vi "move-delayline-eventSD.vi"(3 "Delay pos (mm)":dbl, 4 "choix cible":u16(ring)=2 items=["definir position", "deplacer relatif", "deplacer absolu"], 6 "deplacement in":refnum<vi>) -> (0 "Delay (ps)":dbl=-0.0, 1 "moved":string, 2 "Delay (mm)":dbl, 5 "deplacement boolean":bool)   [LabVIEW 2015]
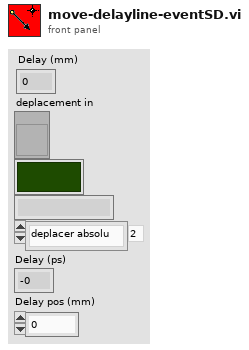
[diagram p1: front panel]
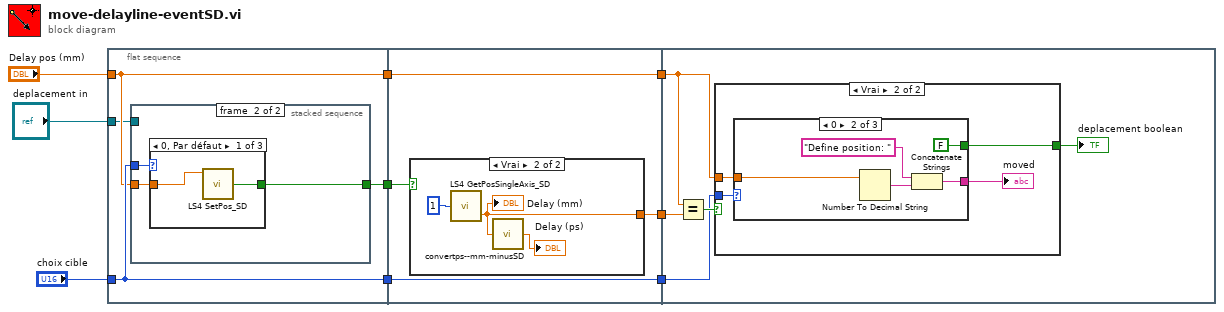
[diagram p0: block diagram]
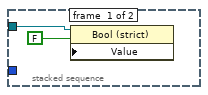
[diagram p2: hidden frame]
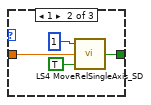
[diagram p3: hidden frame]
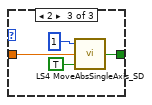
[diagram p4: hidden frame]
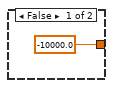
[diagram p5: hidden frame]
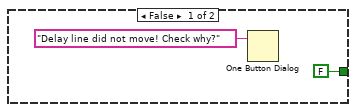
[diagram p6: hidden frame]
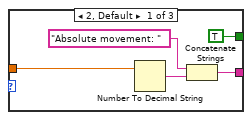
[diagram p7: hidden frame]
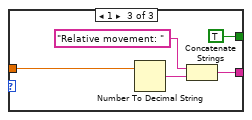
[diagram p8: hidden frame]
diagram:
  n1 = flat-sequence {
    tunnel: "choix cible" -> [w13]
    tunnel: [w13] -> w6
    tunnel: "Delay pos (mm)" -> [w12]
    tunnel: [w12] -> w5
    tunnel: "deplacement in" -> [w10]
    tunnel: [w11] -> w4
    tunnel: w6 -> [w30]
    tunnel: [w30] -> w3
    tunnel: w5 -> [w29]
    tunnel: [w29] -> w2
    tunnel: w4 -> [w32]
    tunnel: [w31] -> w1
    tunnel: w3 -> [w38]
    tunnel: w2 -> [w37]
    tunnel: w1 -> [w39]
    frame #0 {
      n2 = stacked-sequence {
        tunnel: [_ w18] -> w11
        tunnel: w12 -> [_ w17]
        tunnel: w13 -> [_ w16]
        tunnel: w10 -> [w14 _]
        frame #0 {
          n3 = property class="Bool (strict)"(reference=w14, "Value"=FALSE ("deplacement boolean")) -> ()  [unwired: 1 in, 2 out]
        }
        frame #1 {
          n4 = case "Structure Condition" shown="0, Par défaut" w16 {
            tunnel: w17 -> [w20 w22 w26]
            tunnel: [w19 w21 w25] -> w18
            frame 0, Default {
              n5 = call "LS4 SetPos_SD.vi"("X"=w20) -> ("Command executed"=w19:bool)  [unwired: 3 in]
            }
            frame 1 {
              n6 = call "LS4 MoveRelSingleAxis_SD.vi"("Wait"=TRUE, "Value"=w22, "Axis"=1) -> ("Command executed"=w21:bool)
            }
            frame 2 {
              n7 = call "LS4 MoveAbsSingleAxis_SD.vi"("Wait"=TRUE, "Value"=w26, "Axis"=1) -> ("Command executed"=w25:bool)
            }
          }
        }
      }
    }
    frame #1 {
      n8 = case shown="Vrai" w32 {
        tunnel: [-10000.0 ("Pos") w34] -> w31
        frame False {
        }
        frame True {
          n9 = call "LS4 GetPosSingleAxis_SD.vi"("Axis"=1) -> ("Pos"=w34:dbl)  [unwired: 1 out]
          "Delay (mm)" <- w34
          n10 = call "convertps--mm-minusSD.vi"("mm"=w34) -> ("ps"=→"Delay (ps)":dbl)
        }
      }
    }
    frame #2 {
      n11 = Equal?(x=w37, y=w39) -> (x = y?=w41:bool)
      n12 = case shown="Vrai" w41 {
        tunnel: w38 -> [_ w47]
        tunnel: [FALSE ("deplacement boolean") w44] -> w40
        tunnel: w37 -> [_ w46]
        frame False {
          n13 = One Button Dialog(message="Delay line did not move! Check why?") -> ()  [unwired: 1 in, 1 out]
        }
        frame True {
          n14 = case shown="0" w47 {
            tunnel: w46 -> [w50 w55 w60]
            tunnel: [w49 w54 w59] -> w45
            tunnel: [TRUE ("deplacement boolean") FALSE ("deplacement boolean") TRUE ("deplacement boolean")] -> w44
            frame 2, Default {
              n15 = Number To Decimal String(number=w50) -> (decimal integer string=w51:string)  [unwired: 1 in]
              n16 = Concatenate Strings("Absolute movement: " ("moved"), w51) -> (w49:string)
            }
            frame 0 {
              n17 = Number To Decimal String(number=w55) -> (decimal integer string=w56:string)  [unwired: 1 in]
              n18 = Concatenate Strings("Define position: " ("moved"), w56) -> (w54:string)
            }
            frame 1 {
              n19 = Number To Decimal String(number=w60) -> (decimal integer string=w61:string)  [unwired: 1 in]
              n20 = Concatenate Strings("Relative movement: " ("moved"), w61) -> (w59:string)
            }
          }
          "moved" <- w45
        }
      }
      "deplacement boolean" <- w40
    }
  }
